vi "About.vi"(8 "error in (no error)":errorcluster) -> (0 "error out":errorcluster)   [LabVIEW 2015]
panel:
  in  "Animation":u16(ring)=9
  # "试验测试系统软件"
  # "QQ:1987747810"
  # "Version: 1.3.2\nCopyright(C)2012\nwanghongbo All rights reserved."
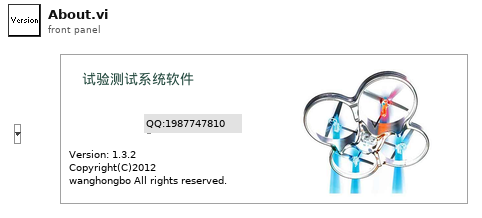
[diagram p1: front panel]
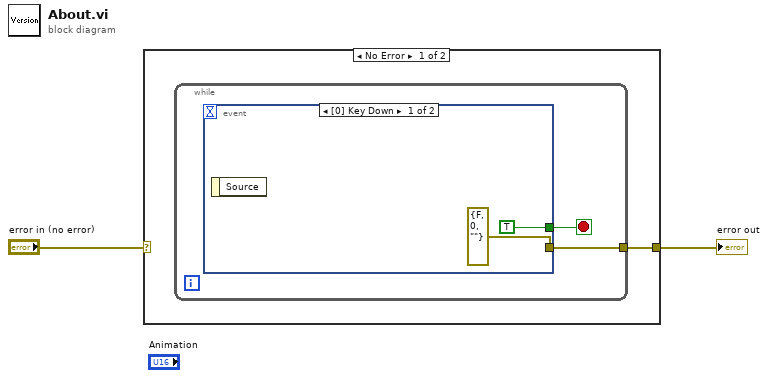
[diagram p0: block diagram]
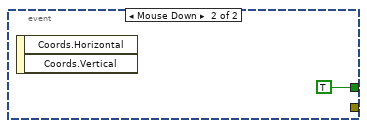
[diagram p2: hidden frame]
diagram:
  n1 = case shown="No Error" "error in (no error)" {
    selector: "error in (no error)" -> [_ w9]
    tunnel: [w3 w9] -> w1
    frame No Error {
      n2 = while {
        tunnel: [w4] -> w3
        stop <- w5 stop-if-true
        n3 = event shown="[0] Key Down" {
          selector: _ -> [_ _]
          dyn-events: _ -> [_ _]
          timeout: _ -> [_ _]
          tunnel: [TRUE ("stop") TRUE ("stop")] -> w5
          tunnel: [errorcluster {"status"=FALSE, "code"=0, "source"=""} ("error out") _] -> w4
          event Key Down {
            n4 = event-data() -> ()  [unwired: 2 out]
          }
          event Mouse Down {
            n5 = event-data() -> ()  [unwired: 3 out]
          }
        }
      }
    }
    frame Error {
    }
  }
  "error out" <- w1
